vi "end.vi"(8 "error in (no error)":errorcluster, 11 "Roda_Filtros in":refnum<class "Roda_Filtros.lvclass">) -> (0 "error out":errorcluster, 3 "Roda_Filtros out":refnum<class "Roda_Filtros.lvclass">)   [LabVIEW 2018, in "Roda_Filtros.lvclass"]
uses:
  Roda_Filtros.lvclass
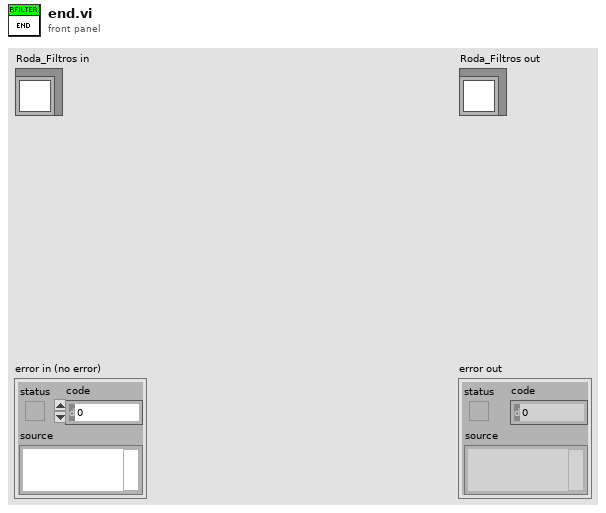
[diagram p1: front panel]
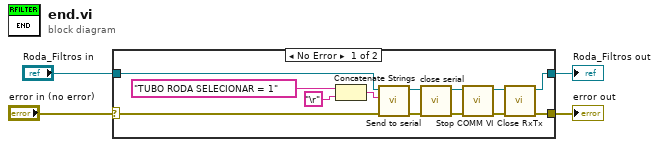
[diagram p0: block diagram]
diagram:
  n1 = case shown="No Error" "error in (no error)" {
    selector: "error in (no error)" -> [w15 w19]
    tunnel: [w6 w19] -> w3
    tunnel: [w7 w18] -> w1
    tunnel: "Roda_Filtros in" -> [w17 w18]
    frame No Error {
      n2 = Concatenate Strings("TUBO RODA SELECIONAR = 1" ("string"), "\r") -> (w13:string)
      n3 = call-dynamic "Send to serial.vi"("error in (no error)"=w15, "message"=w13, "Roda_Filtros in"=w17) -> ("error out"=w14:errorcluster, "Roda_Filtros out"=w16:refnum<class "Roda_Filtros.lvclass">)  [unwired: 7 in]
      n4 = call-dynamic "close serial.vi"("error in (no error)"=w14, "Roda_Filtros in"=w16) -> ("error out"=w9:errorcluster, "Roda_Filtros out"=w10:refnum<class "Roda_Filtros.lvclass">)  [unwired: 8 in]
      n5 = call "Stop COMM VI.vi"("error in (no error)"=w9, "Roda_Filtros in"=w10) -> ("error out"=w5:errorcluster, "Roda_Filtros out"=w8:refnum<class "Roda_Filtros.lvclass">)  [unwired: 8 in]
      n6 = call "Close RxTx.vi"("error in (no error)"=w5, "Roda_Filtros in"=w8) -> ("error out"=w6:errorcluster, "Roda_Filtros out"=w7:refnum<class "Roda_Filtros.lvclass">)  [unwired: 8 in]
    }
    frame Error {
    }
  }
  "error out" <- w3
  "Roda_Filtros out" <- w1
